vi "Autonomous Independent Backup That Doesn't Work.vi"() -> ()   [LabVIEW 2016]
doc: "This VI is called when autonomous begins, and will automatically be terminated when autonomous ends. You can carry out timed or sensor driven robot movement independently without needing to return to the caller."
uses:
  <vilib>/Rock Robotics/Network Tables/NT Read String.vi
panel:
  out "Done With Both":bool
  out "Done With Left":bool
  out "Done With Right":bool
  in  "Array":T1(array[cluster])=[{"Right"=-0.5, "Left"=-0.5, "Sam"=-102.0, "Right Encoder"=-102.0, "Feeder"=0.0, "Shootér"=0.0, "Shootér Encoder"=0.0, "Right Comparison"=enum."Less", "Left Comparison"=enum."Less"}, {"Right"=-0.3, "Left"=0.3, "Sam"=-93.90310397, "Right Encoder"=-110.09689603, "Feeder"=0.0, "Shootér"=0.0, "Shootér Encoder"=0.0, "Right Comparison"=enum."Less", "Left Comparison"=enum."Greater"}, {"Right"=-0.5, "Left"=-0.5, "Sam"=9.9031, "Right Encoder"=-26.09689603, "Feeder"=0.0, "Shootér"=0.0, "Shootér Encoder"=0.0, "Right Comparison"=enum."Greater", "Left Comparison"=enum."Greater"}, {"Right"=0.3, "Left"=-0.3, "Sam"=-1.8062, "Right Encoder"=-34.1938, "Feeder"=0.0, "Shootér"=0.0, "Shootér Encoder"=0.0, "Right Comparison"=enum."Greater", "Left Comparison"=enum."Greater"}, {"Right"=0.0, "Left"=0.0, "Sam"=0.0, "Right Encoder"=0.0, "Feeder"=1.0, "Shootér"=0.7, "Shootér Encoder"=0.0, "Right Comparison"=enum."Zero", "Left Comparison"=enum."Zero"}]
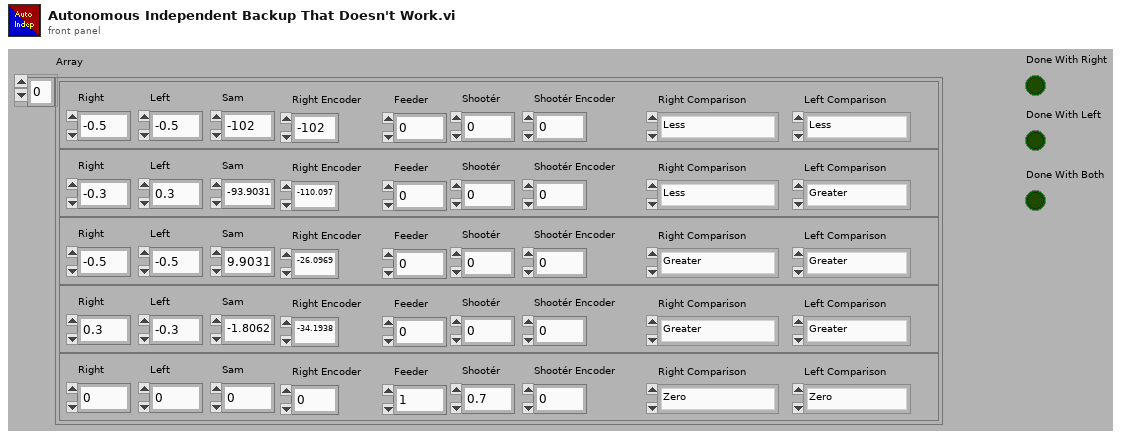
[diagram p1: front panel]
types:
  T1 = cluster{"Right":dbl, "Left":dbl, "Sam":dbl, "Right Encoder":dbl, "Feeder":dbl, "Shootér":dbl, "Shootér Encoder":dbl, "Right Comparison":enum16{"Greater", "Less", "Zero"}, "Left Comparison":enum16{"Greater", "Less", "Zero"}}[]
  T2 = typedef "WPI_EncoderDevRef.ctl" = cluster{"DevStatus":errorcluster, "EncoderIndex":T3, "CounterIndex":T4, "DistancePerCount":dbl, "Decoding Type":T5}
  T3 = typedef "FPGA_EncoderIdx.ctl" = enum8{"Enc 0", "Enc 1", "Enc 2", "Enc 3", "Enc 4", "Enc 5", "Enc 6", "Enc 7", "Invalid"}
  T4 = typedef "FPGA_CounterCtrSystemIndex.ctl" = enum8{"Ctr 0", "Ctr 1", "Ctr 2", "Ctr 3", "Ctr 4", "Ctr 5", "Ctr 6", "Ctr 7", "Invalid"}
  T5 = typedef "WPI_EncoderType.ctl" = enum16{"1x", "2x", "4x"}
  T6 = typedef "WPI_MotorControlDeviceRef.ctl" = cluster{"DeviceStatus":errorcluster, "Type":T7, "PWM":cluster{"PWM Channel":T8, "DeadBand":T9}, "CAN":cluster{"Device Number":u8, "SetOutput VI Ref":variant, "GetOutput VI Ref":variant, "Enable VI Ref":variant, "Disable VI Ref":variant, "Data":variant}, "Invert":bool}
  T7 = typedef "WPI_MotorControlType.ctl" = enum16{"PWM", "CAN"}
  T8 = typedef "FPGA_DIOPWMChannel.ctl" = enum8{"PWM 0", "PWM 1", "PWM 2", "PWM 3", "PWM 4", "PWM 5", "PWM 6", "PWM 7", "PWM 8", "PWM 9", "PWM MXP 0", "PWM MXP 1", "PWM MXP 2", "PWM MXP 3", "PWM MXP 4", "PWM MXP 5", "PWM MXP 6", "PWM MXP 7", "PWM MXP 8", "PWM MXP 9", "Invalid"}
  T9 = typedef "WPI_PWMDeadband.ctl" = cluster{"Name":string, "maxPositivePwm":i32, "minPositivePwm":i32, "centerPwm":i32, "maxNegativePwm":i32, "minNegativePwm":i32, "angularRange":u16}
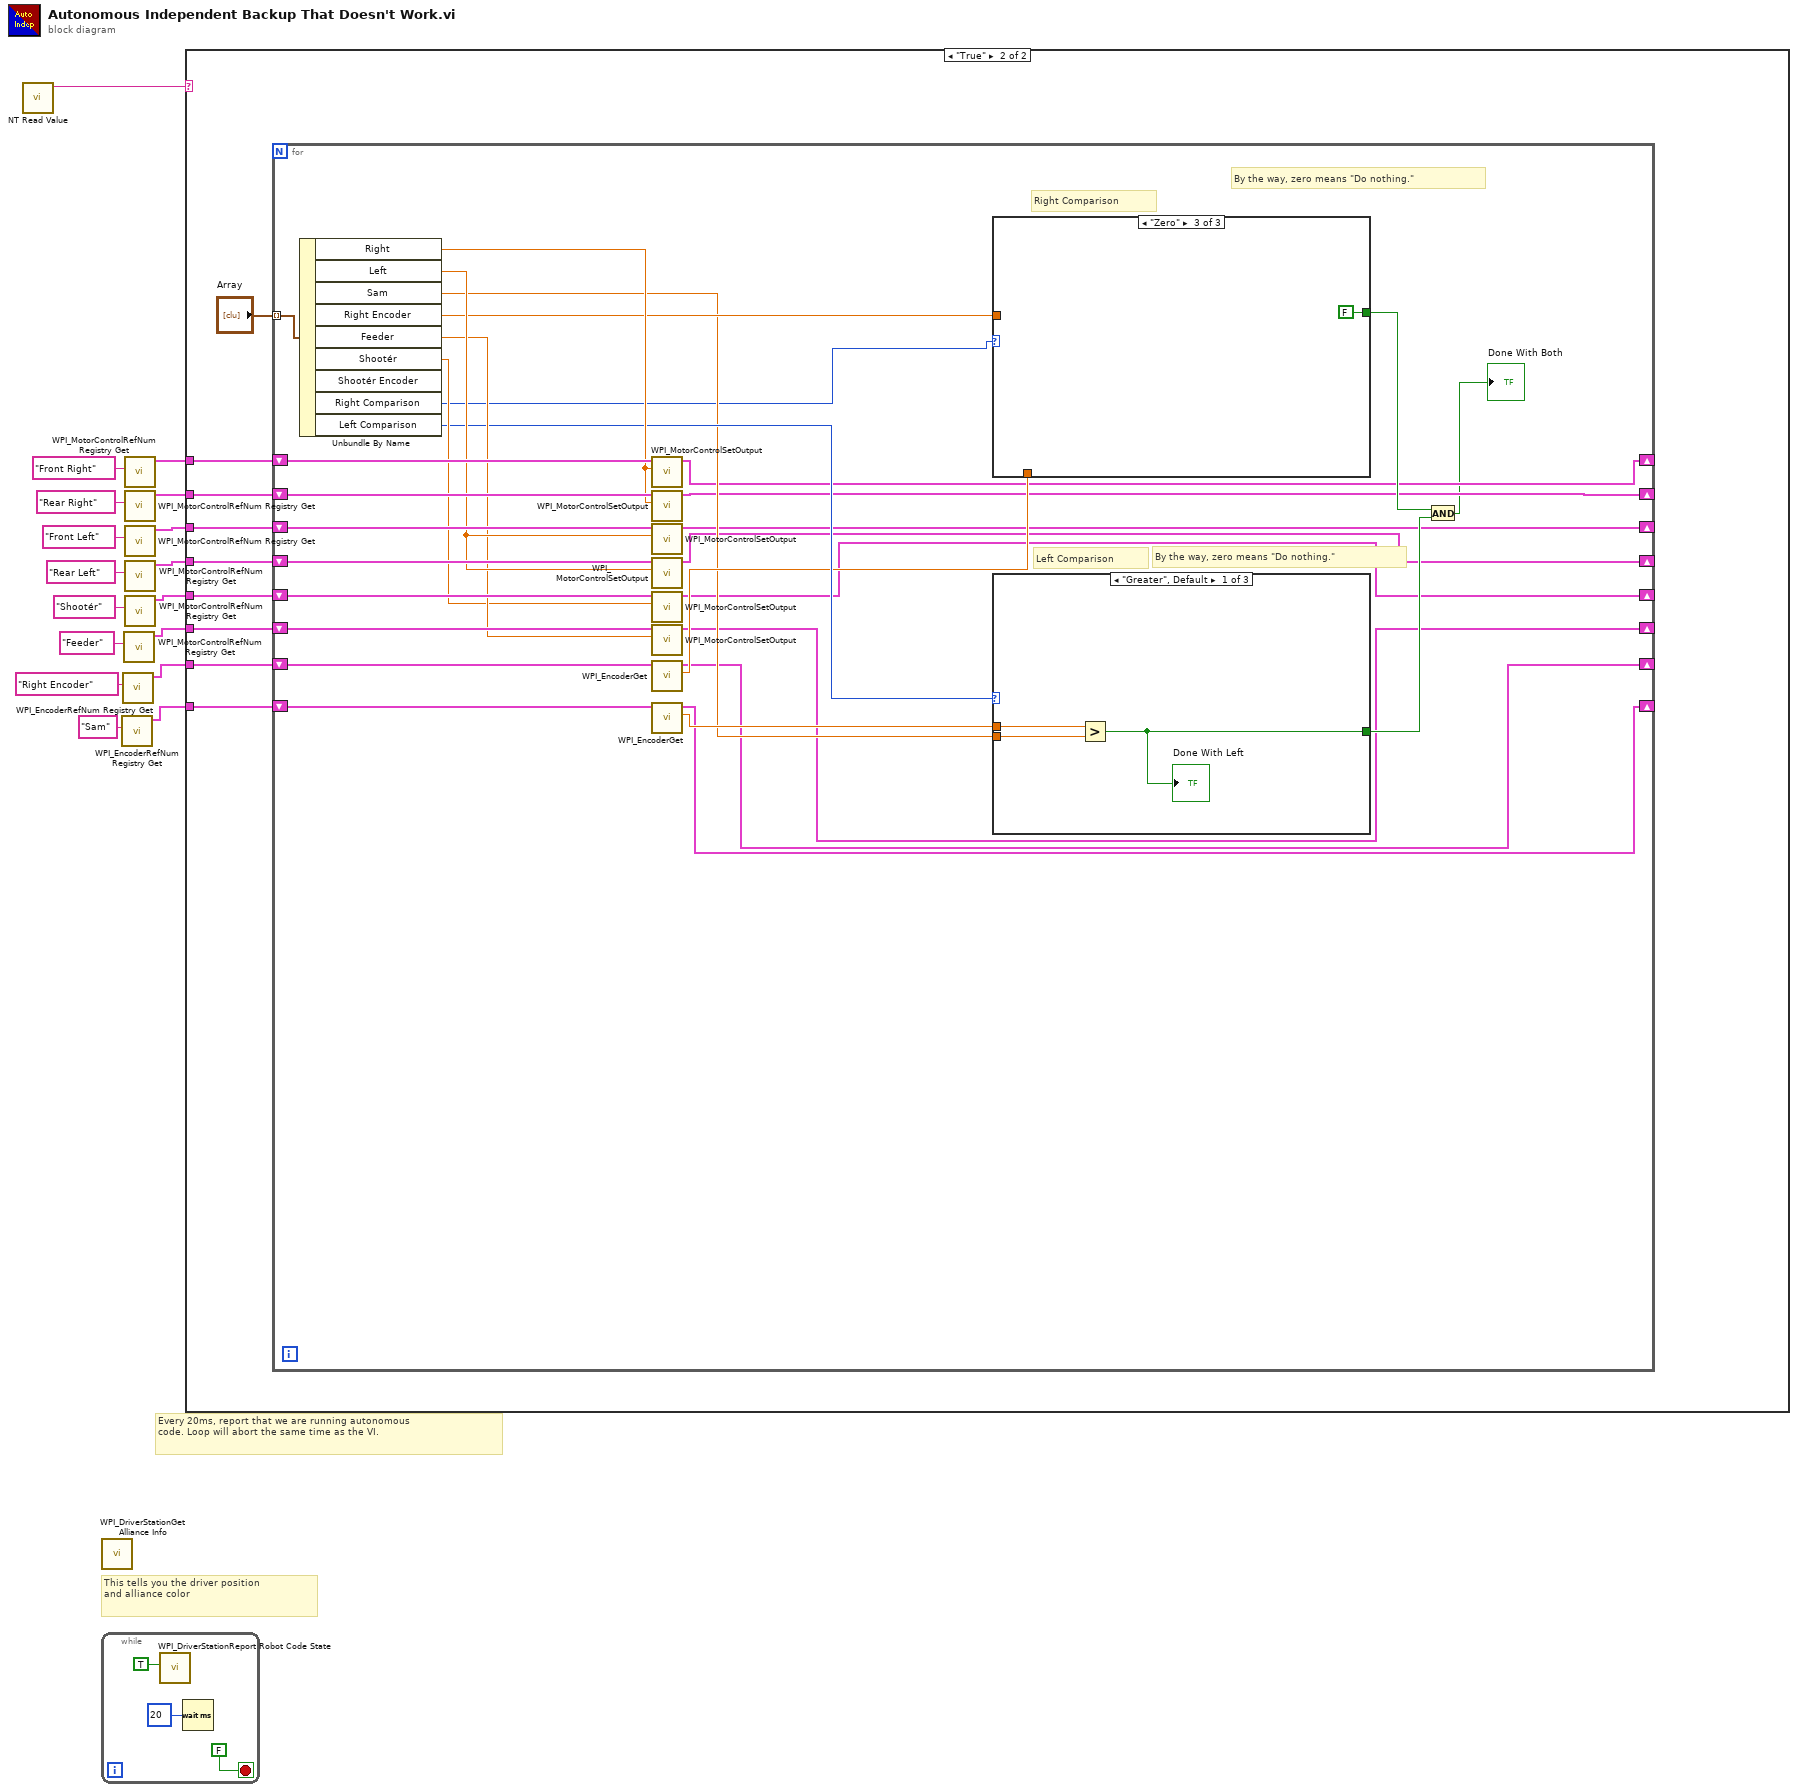
[diagram p0: block diagram]
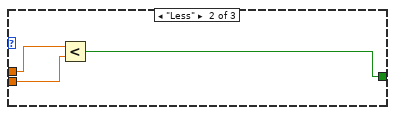
[diagram p3: hidden frame]
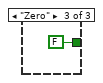
[diagram p4: hidden frame]
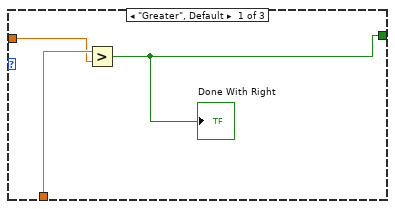
[diagram p5: hidden frame]
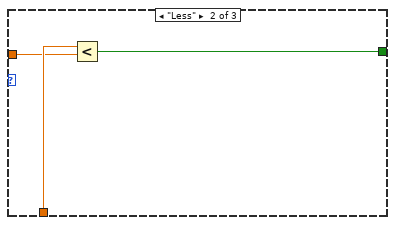
[diagram p6: hidden frame]
diagram:
  # "Every 20ms, report that we are running autonomous\ncode. Loop will abort the same time as the VI."
  # "This tells you the driver position\nand alliance color"
  n1 = call-poly <vilib>:"NT Read Value.vi"() -> ("String"=w17:string)  [unwired: 10 in, 1 out]
  n2 = call <vilib>:"WPI_DriverStationGet Alliance Info.vi"() -> ()  [unwired: 12 out]
  n3 = while {
    stop <- FALSE stop-if-true
    n4 = call <vilib>:"WPI_DriverStationReport Robot Code State.vi"("Autonomous"=TRUE) -> ()  [unwired: 10 in, 1 out]
    n5 = Wait (ms)(milliseconds to wait=u32 20) -> ()  [unwired: 1 out]
  }
  n6 = call <vilib>:"WPI_EncoderRefNum Registry Get.vi"("refnum name"="Sam") -> ("EncoderDevRef"=w1:T2)  [unwired: 9 in, 1 out]
  n7 = call <vilib>:"WPI_EncoderRefNum Registry Get.vi"("refnum name"="Right Encoder") -> ("EncoderDevRef"=w3:T2)  [unwired: 9 in, 1 out]
  n8 = call <vilib>:"WPI_MotorControlRefNum Registry Get.vi"("refnum name"="Feeder") -> ("MotorControlDevRef"=w5:T6)  [unwired: 9 in, 1 out]
  n9 = call <vilib>:"WPI_MotorControlRefNum Registry Get.vi"("refnum name"="Front Right") -> ("MotorControlDevRef"=w10:T6)  [unwired: 9 in, 1 out]
  n10 = call <vilib>:"WPI_MotorControlRefNum Registry Get.vi"("refnum name"="Rear Right") -> ("MotorControlDevRef"=w9:T6)  [unwired: 9 in, 1 out]
  n11 = call <vilib>:"WPI_MotorControlRefNum Registry Get.vi"("refnum name"="Front Left") -> ("MotorControlDevRef"=w8:T6)  [unwired: 9 in, 1 out]
  n12 = call <vilib>:"WPI_MotorControlRefNum Registry Get.vi"("refnum name"="Rear Left") -> ("MotorControlDevRef"=w7:T6)  [unwired: 9 in, 1 out]
  n13 = call <vilib>:"WPI_MotorControlRefNum Registry Get.vi"("refnum name"="Shootér") -> ("MotorControlDevRef"=w6:T6)  [unwired: 9 in, 1 out]
  n14 = case shown="\"True\"" w17 {
    tunnel: w10 -> [_ w28]
    tunnel: w9 -> [_ w27]
    tunnel: w8 -> [_ w26]
    tunnel: w7 -> [_ w25]
    tunnel: w6 -> [_ w24]
    tunnel: w5 -> [_ w23]
    tunnel: w3 -> [_ w22]
    tunnel: w1 -> [_ w21]
    frame "False", Default {
    }
    frame "True" {
      n15 = for {
        tunnel: "Array" -> [w59] mode=indexing
        shift-right: [w39] -> _
        shift-left: w28 -> [w58]
        shift-right: [w38] -> _
        shift-left: w27 -> [w57]
        shift-right: [w37] -> _
        shift-left: w26 -> [w56]
        shift-right: [w36] -> _
        shift-left: w25 -> [w55]
        shift-right: [w35] -> _
        shift-left: w24 -> [w54]
        shift-right: [w34] -> _
        shift-left: w23 -> [w53]
        shift-right: [w33] -> _
        shift-left: w22 -> [w48]
        shift-right: [w32] -> _
        shift-left: w21 -> [w46]
        # "By the way, zero means \"Do nothing.\""
        # "By the way, zero means \"Do nothing.\""
        # "Left Comparison"
        # "Right Comparison"
        n16 = Unbundle By Name(w59) -> ("Right"=w52:dbl, "Left"=w51:dbl, "Sam"=w42:dbl, "Right Encoder"=w43:dbl, "Feeder"=w50:dbl, "Shootér"=w49:dbl, "Right Comparison"=w30:enum16{"Greater", "Less", "Zero"}, "Left Comparison"=w47:enum16{"Greater", "Less", "Zero"})  [unwired: 1 out]
        n17 = call <vilib>:"WPI_MotorControlSetOutput.vi"("Output"=w52, "MotorControlDevRef"=w58) -> ("MotorControlDevRef"=w39:T6)  [unwired: 7 in, 2 out]
        n18 = call <vilib>:"WPI_MotorControlSetOutput.vi"("Output"=w52, "MotorControlDevRef"=w57) -> ("MotorControlDevRef"=w38:T6)  [unwired: 7 in, 2 out]
        n19 = call <vilib>:"WPI_MotorControlSetOutput.vi"("Output"=w51, "MotorControlDevRef"=w56) -> ("MotorControlDevRef"=w37:T6)  [unwired: 7 in, 2 out]
        n20 = call <vilib>:"WPI_MotorControlSetOutput.vi"("Output"=w51, "MotorControlDevRef"=w55) -> ("MotorControlDevRef"=w36:T6)  [unwired: 7 in, 2 out]
        n21 = call <vilib>:"WPI_MotorControlSetOutput.vi"("Output"=w49, "MotorControlDevRef"=w54) -> ("MotorControlDevRef"=w35:T6)  [unwired: 7 in, 2 out]
        n22 = call <vilib>:"WPI_MotorControlSetOutput.vi"("Output"=w50, "MotorControlDevRef"=w53) -> ("MotorControlDevRef"=w34:T6)  [unwired: 7 in, 2 out]
        n23 = call <vilib>:"WPI_EncoderGet.vi"("EncoderDevRef"=w48) -> ("Distance"=w45:dbl, "EncoderDevRef"=w33:T2)  [unwired: 5 in, 4 out]
        n24 = call <vilib>:"WPI_EncoderGet.vi"("EncoderDevRef"=w46) -> ("Distance"=w44:dbl, "EncoderDevRef"=w32:T2)  [unwired: 5 in, 4 out]
        n25 = case shown="\"Zero\"" w30 {
          tunnel: w45 -> [w69 w72 _]
          tunnel: w43 -> [w68 w71 _]
          tunnel: [w67 w70 FALSE] -> w41
          frame "Greater", Default {
            n26 = Greater?(x=w69, y=w68) -> (0:w67:bool)
            "Done With Right" <- w67
          }
          frame "Less" {
            n27 = Less?(x=w72, y=w71) -> (x < y?=w70:bool)
          }
          frame "Zero" {
          }
        }
        n28 = case shown="\"Greater\", Default" w47 {
          tunnel: w44 -> [w62 w65 _]
          tunnel: w42 -> [w61 w64 _]
          tunnel: [w60 w63 FALSE] -> w40
          frame "Greater", Default {
            n29 = Greater?(x=w62, y=w61) -> (0:w60:bool)
            "Done With Left" <- w60
          }
          frame "Less" {
            n30 = Less?(x=w65, y=w64) -> (x < y?=w63:bool)
          }
          frame "Zero" {
          }
        }
        n31 = And(x=w41, y=w40) -> (x .and. y?=→"Done With Both":bool)
      }
    }
  }
